vi "PerformanceTest_Create.vi"(8 "error in (no error)":errorcluster, 11 "reference in":refnum<class "PerformanceTest.lvclass">) -> (0 "error out":errorcluster, 3 "reference out":refnum<class "PerformanceTest.lvclass">)   [LabVIEW 2018, in "PerformanceTest.lvclass"]
uses:
  PerformanceTest.lvclass
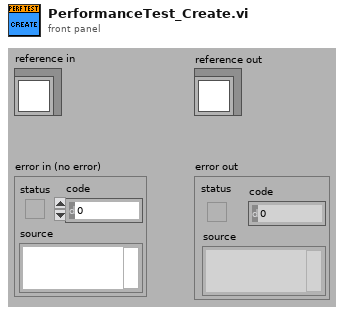
[diagram p1: front panel]
types:
  T1 = typedef "ParentMath.lvclass/ObjectAttributes.ctl" = cluster{"Value":dbl}
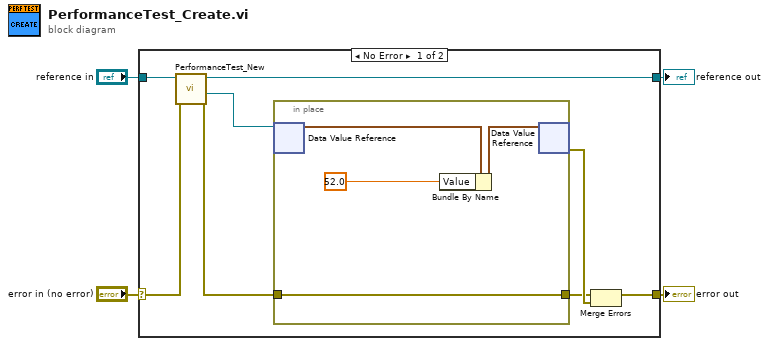
[diagram p0: block diagram]
diagram:
  n1 = case shown="No Error" "error in (no error)" {
    selector: "error in (no error)" -> [w6 w18]
    tunnel: [w8 w18] -> w3
    tunnel: "reference in" -> [w7 w17]
    tunnel: [w12 w17] -> w1
    frame No Error {
      n2 = call "PerformanceTest_New.vi"("error in (no error)"=w6, "reference in"=w7) -> ("error out"=w10:errorcluster, "DVRRefOut"=w5:refnum<data-value>, "reference out"=w12:refnum<class "PerformanceTest.lvclass">)  [unwired: 6 in, 1 out]
      n3 = in-place {
        in-place-border: w10 -> [w14]
        in-place-border: [w14] -> w9
        n4 = in-place-dvr #1(w5) -> (w15:T1)  [unwired: 1 out]
        n5 = Bundle By Name(cluster=w15, "Value"=52.0) -> (w16:T1)
        n6 = in-place-dvr #1(w16) -> (w11:errorcluster)  [unwired: 1 out]
      }
      n7 = Merge Errors(w9, w11) -> (w8:errorcluster)
    }
    frame Error {
      # "VI-TechBaseTemplate_Simple_4x4x4"
    }
  }
  "error out" <- w3
  "reference out" <- w1
